vi "Gen_Channels.vi"() -> (3 "number":u64)   [LabVIEW 2023]
uses:
  <vilib>/numeric/Random Number (Range) U64.vi
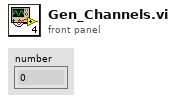
[diagram p1: front panel]
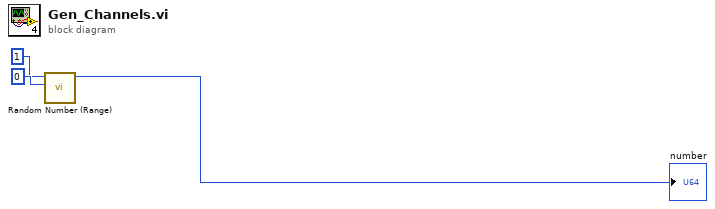
[diagram p0: block diagram]
diagram:
  n1 = call-poly <vilib>:"Random Number (Range).vi"("lower bound (0)"=u64 0, "upper bound (100)"=u64 1) -> ("number"=→"number":u64)  [unwired: 9 in]
